vi "Abort Single Point Load-Single.vi"(8 "error in":errorcluster, 11 "Abort Single Point - Single":T1) -> (0 "error out":errorcluster)   [LabVIEW 2021]
doc: "Abort the single point. In case of error resets the device."
uses:
  controls/Abort Single Point-Single.ctl
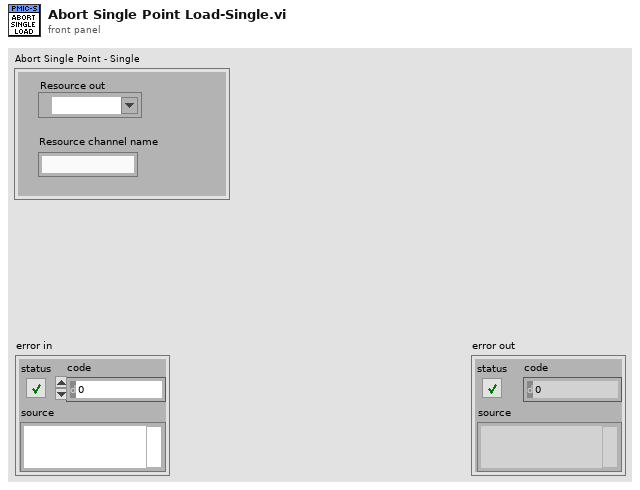
[diagram p1: front panel]
types:
  T1 = typedef "Abort Single Point-Single.ctl" = cluster{"Resource out":refnum<k15>, "Resource channel name":string}
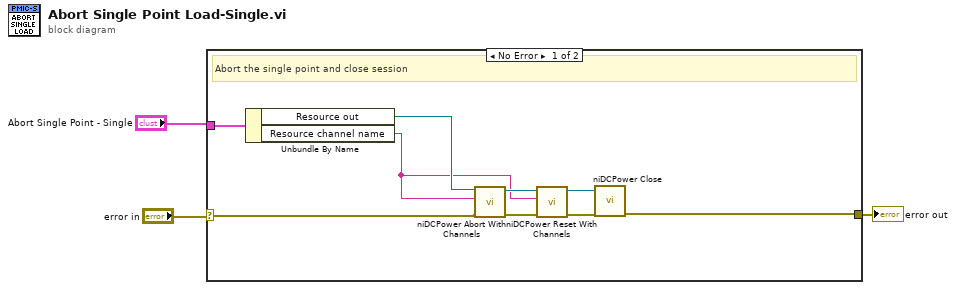
[diagram p0: block diagram]
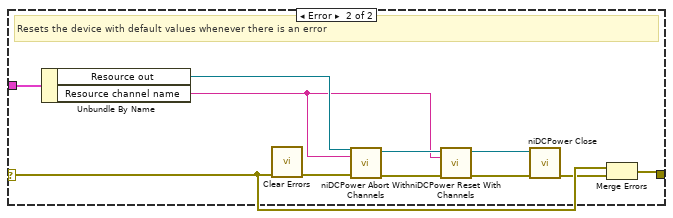
[diagram p2: hidden frame]
diagram:
  n1 = case shown="No Error" "error in" {
    selector: "error in" -> [w9 w15]
    tunnel: "Abort Single Point - Single" -> [w12 w23]
    tunnel: [w10 w13] -> w1
    frame No Error {
      # "Abort the single point and close session"
      n2 = Unbundle By Name(w12) -> ("Resource out"=w11:refnum<k15>, "Resource channel name"=w4:string)
      n3 = call <instrlib>:"niDCPower Abort With Channels.vi"("error in (no error)"=w9, "channel name"=w4, "instrument handle"=w11) -> ("error out"=w8:errorcluster, "instrument handle out"=w5:refnum<k15>)  [unwired: 7 in]
      n4 = call <instrlib>:"niDCPower Reset With Channels.vi"("error in (no error)"=w8, "channel name"=w4, "instrument handle"=w5) -> ("error out"=w7:errorcluster, "instrument handle out"=w6:refnum<k15>)  [unwired: 7 in]
      n5 = call <instrlib>:"niDCPower Close.vi"("error in (no error)"=w7, "instrument handle"=w6) -> ("error out"=w10:errorcluster)  [unwired: 9 in]
    }
    frame Error {
      # "Resets the device with default values whenever there is an error"
      n6 = Unbundle By Name(w23) -> ("Resource out"=w18:refnum<k15>, "Resource channel name"=w17:string)
      n7 = call <vilib>:"Clear Errors.vi"("error in (no error)"=w15) -> ("error out"=w16:errorcluster)  [unwired: 5 in, 1 out]
      n8 = call <instrlib>:"niDCPower Abort With Channels.vi"("error in (no error)"=w16, "channel name"=w17, "instrument handle"=w18) -> ("error out"=w22:errorcluster, "instrument handle out"=w21:refnum<k15>)  [unwired: 7 in]
      n9 = call <instrlib>:"niDCPower Reset With Channels.vi"("error in (no error)"=w22, "channel name"=w17, "instrument handle"=w21) -> ("error out"=w20:errorcluster, "instrument handle out"=w19:refnum<k15>)  [unwired: 7 in]
      n10 = call <instrlib>:"niDCPower Close.vi"("error in (no error)"=w20, "instrument handle"=w19) -> ("error out"=w14:errorcluster)  [unwired: 9 in]
      n11 = Merge Errors(w15, w14) -> (w13:errorcluster)
    }
  }
  "error out" <- w1
